vi "close.vi"(8 "error in (no error)":errorcluster, 11 "DeviceRefnum":u64) -> (0 "error out":errorcluster, 2 "function return":i32)   [LabVIEW 2015, in "rtlsdr.lvlib"]
doc: "Closes the RTLSDR resource.\nIf this is not called upon terminating the application, the resource remains in memory. It will not be possible to open the resource again unless the rtlsdr is undplugged and replugged, or the system is restarted."
uses:
  rtlsdr.lvlib
  rtlsdr/rtlsdr.dll
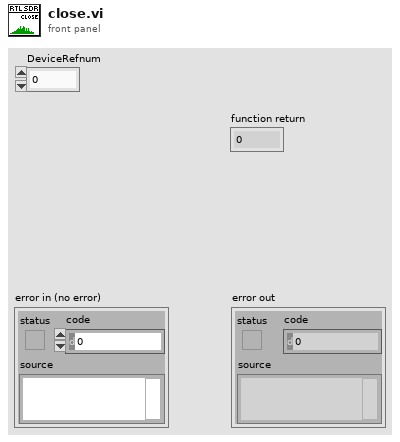
[diagram p1: front panel]
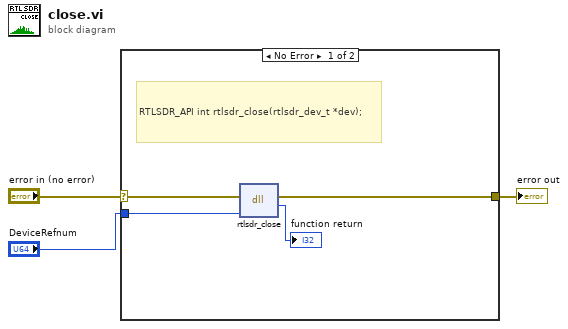
[diagram p0: block diagram]
diagram:
  n1 = case shown="No Error" "error in (no error)" {
    selector: "error in (no error)" -> [w4 w8]
    tunnel: [w5 w8] -> w3
    tunnel: "DeviceRefnum" -> [w7 _]
    frame No Error {
      # "RTLSDR_API int rtlsdr_close(rtlsdr_dev_t *dev);"
      n2 = dll-call lib="C:/Users/TheDoctor/Documents/Projects/Labview Libraries/rtlsdr/rtlsdr.dll" fn="rtlsdr_close"(error in=w4, "DeviceRefnum"=w7) -> (error out=w5:errorcluster, "return type"=→"function return":i32)  [unwired: 3 in, 1 out]
    }
    frame Error {
    }
  }
  "error out" <- w3
